vi "Apply_New_Window_Center.vi"(7 "Chan# (only Channel 0 works now)":i8, 9 "ResetTrig":bool, 10 "User Trig":T2, 11 "FeedbackTrig":T1) -> (2 "AllWindows out":T2)   [LabVIEW 2021]
doc: "Use this VI to update the window center.\nWhen we trigger (on the high side or the low side of the trigger window), use the triggering signal value as the new window center.\nLuke 11-18-2022"
uses:
  Host/Clusts/AllWindowsClust.ctl
  Host/Clusts/ChannelWindowClust.ctl
  Controls/Clust/Update_Trigger_Center.ctl
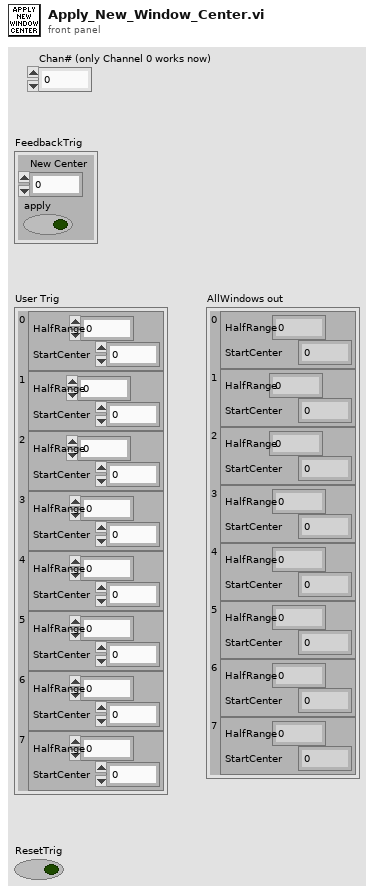
[diagram p1: front panel]
types:
  T1 = typedef "Update_Trigger_Center.ctl" = cluster{"New Center":fxp<+/-,18,5>, "apply":bool}
  T2 = typedef "AllWindowsClust.ctl" = cluster{"0":T3, "1":T3, "2":T3, "3":T3, "4":T3, "5":T3, "6":T3, "7":T3}
  T3 = typedef "ChannelWindowClust.ctl" = cluster{"HalfRange":fxp<+/-,18,5>, "StartCenter":fxp<+/-,18,5>}
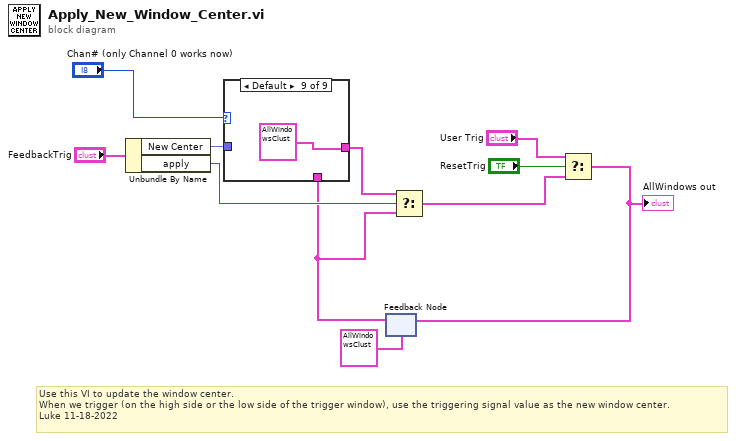
[diagram p0: block diagram]
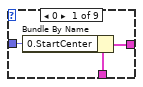
[diagram p2: hidden frame]
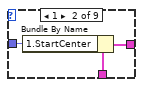
[diagram p3: hidden frame]
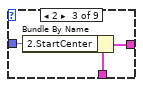
[diagram p4: hidden frame]
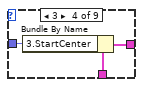
[diagram p5: hidden frame]
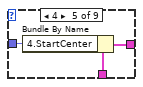
[diagram p6: hidden frame]
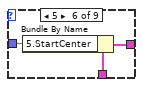
[diagram p7: hidden frame]
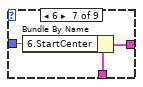
[diagram p8: hidden frame]
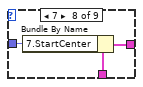
[diagram p9: hidden frame]
diagram:
  # "Use this VI to update the window center.\nWhen we trigger (on the high side or the low side of the trigger window), use the triggering signal value as the new window center.\nLuke 11-18-2022"
  n1 = Unbundle By Name("FeedbackTrig") -> ("New Center"=w9:fxp<+/-,18,5>, "apply"=w8:bool)
  n2 = feedback #1(T2 {"0"={"HalfRange"=0.0, "StartCenter"=0.0}, "1"={"HalfRange"=0.0, "StartCenter"=0.0}, "2"={"HalfRange"=0.0, "StartCenter"=0.0}, "3"={"HalfRange"=0.0, "StartCenter"=0.0}, "4"={"HalfRange"=0.0, "StartCenter"=0.0}, "5"={"HalfRange"=0.0, "StartCenter"=0.0}, "6"={"HalfRange"=0.0, "StartCenter"=0.0}, "7"={"HalfRange"=0.0, "StartCenter"=0.0}} ("User Trig")) -> (w3:T2)
  n3 = case shown="Default" "Chan# (only Channel 0 works now)" {
    tunnel: [w14 w17 w20 w23 w26 w29 w32 w35 T2 {"0"={"HalfRange"=0.0, "StartCenter"=0.0}, "1"={"HalfRange"=0.0, "StartCenter"=0.0}, "2"={"HalfRange"=0.0, "StartCenter"=0.0}, "3"={"HalfRange"=0.0, "StartCenter"=0.0}, "4"={"HalfRange"=0.0, "StartCenter"=0.0}, "5"={"HalfRange"=0.0, "StartCenter"=0.0}, "6"={"HalfRange"=0.0, "StartCenter"=0.0}, "7"={"HalfRange"=0.0, "StartCenter"=0.0}} ("User Trig Default")] -> w11
    tunnel: w9 -> [w13 w16 w19 w22 w25 w28 w31 w34 _]
    tunnel: w3 -> [w12 w15 w18 w21 w24 w27 w30 w33 _]
    frame 0 {
      n4 = Bundle By Name(cluster=w12, "0.StartCenter"=w13) -> (w14:T2)
    }
    frame 1 {
      n5 = Bundle By Name(cluster=w15, "1.StartCenter"=w16) -> (w17:T2)
    }
    frame 2 {
      n6 = Bundle By Name(cluster=w18, "2.StartCenter"=w19) -> (w20:T2)
    }
    frame 3 {
      n7 = Bundle By Name(cluster=w21, "3.StartCenter"=w22) -> (w23:T2)
    }
    frame 4 {
      n8 = Bundle By Name(cluster=w24, "4.StartCenter"=w25) -> (w26:T2)
    }
    frame 5 {
      n9 = Bundle By Name(cluster=w27, "5.StartCenter"=w28) -> (w29:T2)
    }
    frame 6 {
      n10 = Bundle By Name(cluster=w30, "6.StartCenter"=w31) -> (w32:T2)
    }
    frame 7 {
      n11 = Bundle By Name(cluster=w33, "7.StartCenter"=w34) -> (w35:T2)
    }
    frame Default {
    }
  }
  n12 = Select(t=w11, s=w8, f=w3) -> (s? t:f=w4:T2)
  n13 = Select(t="User Trig", s="ResetTrig", f=w4) -> (s? t:f=w2:T2)
  "AllWindows out" <- w2
  n14 = feedback-in #1(w2) -> ()
